vi "Run Filter.vi"(8 "error in (no error)":errorcluster, 10 "resource entries in":T1[](array[typedef]), 11 "Datatype Filter in":refnum<class "Datatype Filter.lvclass">) -> (0 "error out":errorcluster, 2 "resource entries out":T1[](array[typedef]))   [LabVIEW 2016, in "Datatype Filter.lvclass"]
uses:
  Datatype Filter.lvclass
  FPGA-Addon/Source/System Explorer/SubVIs/fpga resource.ctl
  FPGA-Addon/Source/System Explorer/SubVIs/Channel Type.ctl
  Datatype Filter.lvclass/Datatype Filter.ctl
  FPGA-Addon/Source/System Explorer/FPGA Addon System Explorer.lvlib
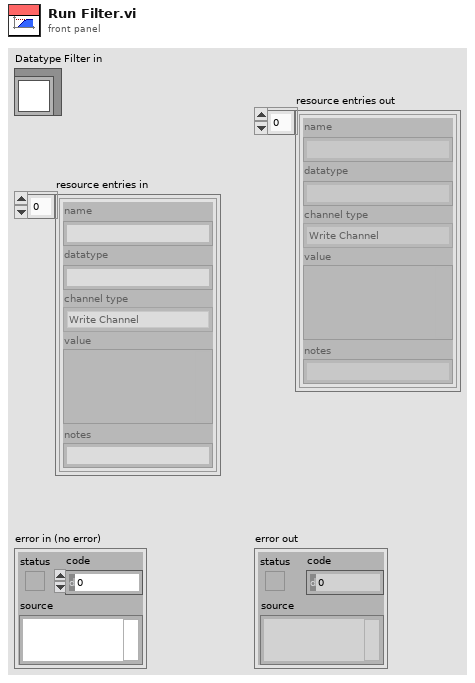
[diagram p1: front panel]
types:
  T1 = typedef "FPGA Addon System Explorer.lvlib/fpga resource.ctl" = cluster{"name":string, "datatype":string, "channel type":T2, "value":variant, "notes":string}
  T2 = typedef "FPGA Addon System Explorer.lvlib/Channel Type.ctl" = enum16{"Write Channel", "Read Channel", "Write Waveform", "Read Waveform"}
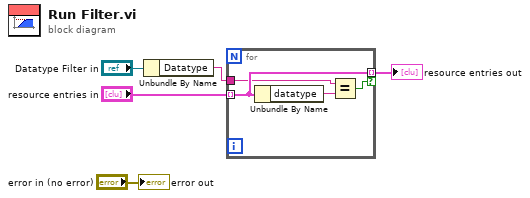
[diagram p0: block diagram]
diagram:
  n1 = Unbundle By Name("Datatype Filter in") -> ("Datatype"=w4:string)
  n2 = for {
    tunnel: w4 -> [w7]
    tunnel: "resource entries in" -> [w9] mode=indexing
    tunnel: [w9] -> w2 mode=indexing if=w6
    n3 = Unbundle By Name(w9) -> ("datatype"=w8:string)
    n4 = Equal?(x=w7, y=w8) -> (x = y?=w6:bool)
  }
  "resource entries out" <- w2
  "error out" <- "error in (no error)"
